vi "WLAN TxP Servo Power.vi"(0 "Instrument Handle In":refnum<k21>, 1 "Selector String":string, 5 "RFSG Session in":refnum<k15>, 7 "WLAN TxP Servo Configuration":T3={"Target TxP Power (dBm)"=0.0, "Tolerance (dB)"=0.05, "Max Number of Iterations"=10}, 9 "Auto Level Configuration":T1={"Enabled"=FALSE, "Measurement Interval (s)"=0.01} {"Measurement Interval (s)" min=1e-06 max=100.0 format="%.2p"}, 11 "error in (no error)":errorcluster) -> (4 "Instrument Handle Out":refnum<k21>, 6 "RFSG Session out":refnum<k15>, 8 "WLAN TxP Servo Power Results":T2, 15 "error out":errorcluster)   [LabVIEW 2016, in "RFmxWLAN.lvlib"]
uses:
  RFmxWLAN.lvlib
  Typedefs/WLAN TxP Servo Configuration.ctl
  Typedefs/WLAN TxP Servo Results.ctl
  Common/SA Auto Level Configuration.ctl
  <vilib>/RFmx/WLAN/mx/RFmxWLAN.llb/RFmxWLAN Select Measurement (Single).vi
  <vilib>/RFmx/WLAN/mx/RFmxWLAN.llb/RFmxWLAN TXP Fetch Measurement.vi
  <resource>/objmgr/RFmxWLAN.rc
  Common/Common.lvlib
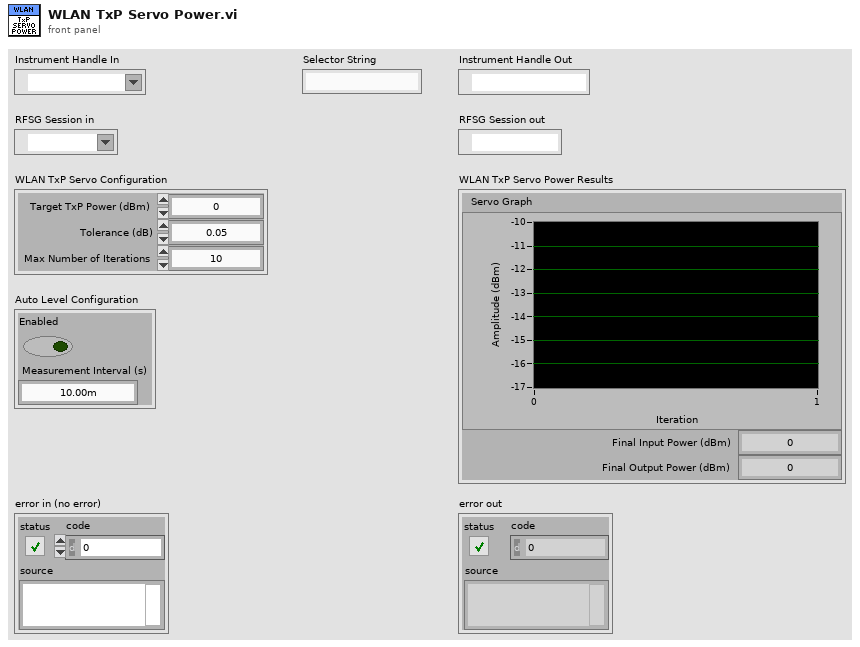
[diagram p1: front panel]
types:
  T1 = typedef "Common.lvlib/SA Auto Level Configuration.ctl" = cluster{"Enabled":bool, "Measurement Interval (s)":dbl}
  T2 = typedef "RFmxWLAN.lvlib/WLAN TxP Servo Results.ctl" = cluster{"Servo Graph":dbl[], "Final Input Power (dBm)":dbl, "Final Output Power (dBm)":dbl}
  T3 = typedef "RFmxWLAN.lvlib/WLAN TxP Servo Configuration.ctl" = cluster{"Target TxP Power (dBm)":dbl, "Tolerance (dB)":dbl, "Max Number of Iterations":i32}
  T4 = enum16{"TXP", "PowerRamp", "DSSSModAcc", "OFDMModAcc", "SEM"}
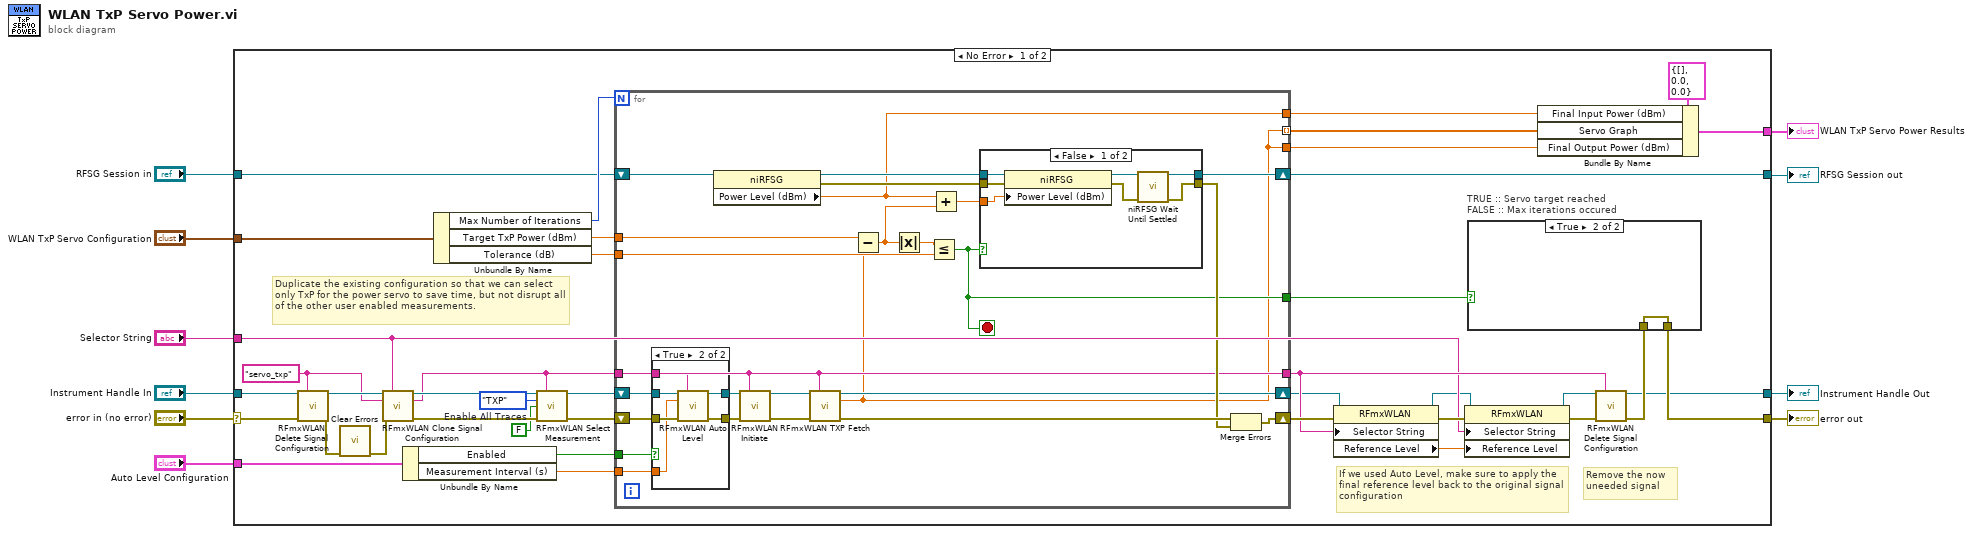
[diagram p0: block diagram]
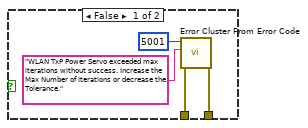
[diagram p4: hidden frame]
diagram:
  n1 = case shown="No Error" "error in (no error)" {
    selector: "error in (no error)" -> [w47 w100]
    tunnel: [w44 w100] -> w10
    tunnel: "Instrument Handle In" -> [w23 w99]
    tunnel: "Selector String" -> [w14 _]
    tunnel: [w39 w99] -> w6
    tunnel: "RFSG Session in" -> [w36 w98]
    tunnel: "WLAN TxP Servo Configuration" -> [w37 _]
    tunnel: [w28 _] -> w3
    tunnel: [w27 w98] -> w2
    tunnel: "Auto Level Configuration" -> [w26 _]
    frame No Error {
      w40 = FALSE  # Enable All Traces
      w21 = "servo_txp" ("New Signal Name")
      # "Remove the now  uneeded signal"
      # "If we used Auto Level, make sure to apply the final reference level back to the original signal configuration"
      # "Duplicate the existing configuration so that we can select only TxP for the power servo to save time, but not disrupt all of the other user enabled measurements."
      n2 = call <vilib>:"RFmxWLAN Delete Signal Configuration.vi"("Instrument Handle In"=w23, "Signal Name"=w21, "error in (no error)"=w47) -> ("Instrument Handle Out"=w22:refnum<k21>, "error out"=w20:errorcluster)  [unwired: 11 in]
      n3 = call <vilib>:"Clear Errors.vi"("error in (no error)"=w20) -> ("error out"=w19:errorcluster)  [unwired: 5 in, 1 out]
      n4 = call <vilib>:"RFmxWLAN Clone Signal Configuration.vi"("Instrument Handle In"=w22, "Old Signal Name"=w14, "New Signal Name"=w21, "error in (no error)"=w19) -> ("Instrument Handle Out"=w43:refnum<k21>, "Selector String Out"=w38:string, "error out"=w49:errorcluster)  [unwired: 9 in]
      n5 = Unbundle By Name(w26) -> ("Enabled"=w25:bool, "Measurement Interval (s)"=w24:dbl)
      n6 = Unbundle By Name(w37) -> ("Max Number of Iterations"=w50:i32, "Target TxP Power (dBm)"=w35:dbl, "Tolerance (dB)"=w34:dbl)
      n7 = call-poly <vilib>:"RFmxWLAN Select Measurement.vi"("Instrument Handle In"=w43, "Selector String"=w38, "Measurement"=T4."TXP", "Enable All Traces"=w40, "error in (no error)"=w49) -> ("Instrument Handle Out"=w42:refnum<k21>, "error out"=w48:errorcluster)  [unwired: 9 in]
      n8 = for {
        N: w50 -> [_]
        tunnel: w38 -> [w55]
        shift-right: [w70] -> w46
        shift-left: w48 -> [w74]
        shift-right: [w67] -> w12
        shift-left: w42 -> [w68]
        tunnel: [w55] -> w17
        shift-right: [w61] -> w27
        shift-left: w36 -> [w64]
        tunnel: w35 -> [w63]
        tunnel: w34 -> [w58]
        tunnel: [w56] -> w33
        tunnel: [w54] -> w31
        tunnel: [w51] -> w30 mode=indexing
        tunnel: [w51] -> w29
        tunnel: w25 -> [w53]
        tunnel: w24 -> [w52]
        stop <- w56 stop-if-true
        n9 = case shown="True" w53 {
          tunnel: [w76 w83] -> w75
          tunnel: w74 -> [w76 w82]
          tunnel: w68 -> [w77 w81]
          tunnel: [w77 w80] -> w66
          tunnel: w55 -> [_ w79]
          tunnel: w52 -> [_ w78]
          frame False {
          }
          frame True {
            n10 = call <vilib>:"RFmxWLAN Auto Level.vi"("Instrument Handle In"=w81, "Selector String"=w79, "Measurement Interval (s)"=w78, "error in (no error)"=w82) -> ("Instrument Handle Out"=w80:refnum<k21>, "error out"=w83:errorcluster)  [unwired: 10 in]
          }
        }
        n11 = property class="niRFSG"(reference=w64) -> (reference out=w62:refnum<k15>, error out=w71:errorcluster, "Power Level (dBm)"=w54:dbl)  [unwired: 1 in]
        n12 = call <vilib>:"RFmxWLAN Initiate.vi"("Instrument Handle In"=w66, "Selector String"=w55, "error in (no error)"=w75) -> ("Instrument Handle Out"=w65:refnum<k21>, "error out"=w72:errorcluster)  [unwired: 10 in, 1 out]
        n13 = call-poly <vilib>:"RFmxWLAN TXP Fetch.vi"("Instrument Handle In"=w65, "Selector String"=w55, "error in (no error)"=w72) -> ("Instrument Handle Out"=w67:refnum<k21>, "Average Power Mean (dBm)"=w51:dbl, "error out"=w73:errorcluster)  [unwired: 9 in, 1 out]
        n14 = Subtract(x=w63, y=w51) -> (x-y=w60:dbl)
        n15 = Absolute Value(x=w60) -> (abs(x)=w57:dbl)
        n16 = Less Or Equal?(x=w57, y=w58) -> (x <= y?=w56:bool)
        n17 = Add(x=w54, y=w60) -> (x+y=w59:dbl)
        n18 = case shown="False" w56 {
          tunnel: w62 -> [w88 w91]
          tunnel: [w84 w91] -> w61
          tunnel: w59 -> [w87 _]
          tunnel: w71 -> [w90 w92]
          tunnel: [w86 w92] -> w69
          frame False {
            n19 = property class="niRFSG"(reference=w88, error in=w90, "Power Level (dBm)"=w87) -> (reference out=w85:refnum<k15>, error out=w89:errorcluster)
            n20 = call <instrlib>:"niRFSG Wait Until Settled.vi"("instrument handle"=w85, "error in"=w89) -> ("instrument handle out"=w84:refnum<k15>, "error out"=w86:errorcluster)  [unwired: 12 in]
          }
          frame True {
          }
        }
        n21 = Merge Errors(w73, w69) -> (w70:errorcluster)
      }
      n22 = property class="RFmxWLAN"(reference=w12, error in=w46, "Selector String"=w17) -> (reference out=w11:refnum<k21>, error out=w18:errorcluster, "Reference Level"=w13:dbl)
      n23 = property class="RFmxWLAN"(reference=w11, error in=w18, "Selector String"=w14, "Reference Level"=w13) -> (reference out=w15:refnum<k21>, error out=w16:errorcluster)
      n24 = Bundle By Name(cluster=T2 {"Servo Graph"=[], "Final Input Power (dBm)"=0.0, "Final Output Power (dBm)"=0.0} ("WLAN TxP Servo Power Results"), "Final Input Power (dBm)"=w31, "Servo Graph"=w30, "Final Output Power (dBm)"=w29) -> (w28:T2)
      n25 = call <vilib>:"RFmxWLAN Delete Signal Configuration.vi"("Instrument Handle In"=w15, "Signal Name"=w17, "error in (no error)"=w16) -> ("Instrument Handle Out"=w39:refnum<k21>, "error out"=w45:errorcluster)  [unwired: 11 in]
      n26 = case "TRUE :: Servo target reached \nFALSE :: Max iterations occured" shown="True" w33 {
        tunnel: w45 -> [w96 w97]
        tunnel: [w95 w97] -> w44
        frame False {
          n27 = call <vilib>:"Error Cluster From Error Code.vi"("error in (no error)"=w96, "error message (\"\")"="WLAN TxP Power Servo exceeded max iterations without success. Increase the Max Number of Iterations or decrease the Tolerance.", "error code (0)"=5001) -> ("error out"=w95:errorcluster)  [unwired: 6 in]
        }
        frame True {
        }
      }
    }
    frame Error {
    }
  }
  "Instrument Handle Out" <- w6
  "error out" <- w10
  "RFSG Session out" <- w2
  "WLAN TxP Servo Power Results" <- w3
